vi "subFD_FXP Modeling & Simu.vi"() -> ()   [LabVIEW 2023]
uses:
  <vilib>/addons/Digital Filter Design/_Objects.llb/DFD Filter Obj.ctl
  <vilib>/addons/Digital Filter Design/_Objects.llb/DFD Filter Coef.ctl
  <vilib>/addons/Digital Filter Design/_Objects.llb/DFD Filter Structure Type Selector.ctl
  <vilib>/addons/Digital Filter Design/_Objects.llb/dfd_Internal Quantization Settings.ctl
  <vilib>/addons/Digital Filter Design/_Objects.llb/dfd_Internal Quantization Srcs.ctl
  <vilib>/addons/Digital Filter Design/_Objects.llb/DFD Coef Norm Type.ctl
  <vilib>/addons/Digital Filter Design/_Objects.llb/DFD Quantization Sources.ctl
  <vilib>/addons/Digital Filter Design/_Objects.llb/DFD FXP Statistics Data.ctl
  <vilib>/addons/Digital Filter Design/FXPModel.llb/DFD FXP Get Quantizer (One).vi
  <vilib>/Utility/VariantDataType/GetNumericFxpInfo.vi
  <vilib>/addons/Digital Filter Design/FXPSim.llb/dfd_Check Input FXP Settings.vi
  <vilib>/addons/Digital Filter Design/FXPSim.llb/dfd_Check SRate Simulation Integer Input.vi
  <vilib>/addons/Digital Filter Design/FXPSim.llb/dfd_FXP Simu.vi
  <vilib>/addons/Digital Filter Design/Process.llb/DFD Filtering (Array).vi
  <vilib>/addons/Digital Filter Design/FXPModel.llb/DFD FXP Set Quantizer (One).vi
  <vilib>/addons/Digital Filter Design/FXPModel.llb/DFD FXP Get Quantizer (All).vi
  <vilib>/addons/Digital Filter Design/FilterLib.llb/DFD Save Filter to File.vi
  <vilib>/addons/Digital Filter Design/FXPSim.llb/SimXnode/DFD FXP Simulation.xnode
  <vilib>/addons/Digital Filter Design/NI_DigFilterLicensed.lvlib
  <vilib>/Analysis/NI_AALBase.lvlib
  <vilib>/Analysis/NI_AALPro.lvlib
  <vilib>/addons/Digital Filter Design/NI_DigFilter_FXP.lvlib
  <vilib>/Utility/VariantDataType/VariantType.lvlib
panel:
  in  "Amplitude":dbl=0.99 min=0.0001 max=1.0 step=0.0001
  in  "Random Input":bool
  in  "Frequency":dbl=1000.1 format="%#_5p Hz"
  in  "Pure Sine Input":bool=TRUE
  in  "Save Filter to File":bool
  in  "Run":bool
  in  "Apply default model?":bool=TRUE
  in  "Delay Quantizer":T1={"source"=1, "wl"=16, "iwl"=1, "o-mode"=0, "q_mode"=0, "signed?"=TRUE} {"q_mode" items=["Nearest", "Truncation"]; "o-mode" items=["Saturation", "Wrap"]; "wl" min=1 max=32 step=1; "source" items=["Coefficient", "Input", "Output", "Multiplicand", "Product", "Sum", "Delay"]}
  in  "Sum Quantizer":T1={"source"=1, "wl"=16, "iwl"=1, "o-mode"=0, "q_mode"=0, "signed?"=TRUE} {"q_mode" items=["Nearest", "Truncation"]; "o-mode" items=["Saturation", "Wrap"]; "wl" min=1 max=32 step=1; "source" items=["Coefficient", "Input", "Output", "Multiplicand", "Product", "Sum", "Delay"]}
  in  "Product Quantizer":T1={"source"=1, "wl"=16, "iwl"=1, "o-mode"=0, "q_mode"=0, "signed?"=TRUE} {"q_mode" items=["Nearest", "Truncation"]; "o-mode" items=["Saturation", "Wrap"]; "wl" min=1 max=32 step=1; "source" items=["Coefficient", "Input", "Output", "Multiplicand", "Product", "Sum", "Delay"]}
  in  "Multiplicand Quantizer":T1={"source"=1, "wl"=16, "iwl"=1, "o-mode"=0, "q_mode"=0, "signed?"=TRUE} {"q_mode" items=["Nearest", "Truncation"]; "o-mode" items=["Saturation", "Wrap"]; "wl" min=1 max=32 step=1; "source" items=["Coefficient", "Input", "Output", "Multiplicand", "Product", "Sum", "Delay"]}
  in  "Output Quantizer":T1={"source"=1, "wl"=16, "iwl"=1, "o-mode"=0, "q_mode"=0, "signed?"=TRUE} {"q_mode" items=["Nearest", "Truncation"]; "o-mode" items=["Saturation", "Wrap"]; "wl" min=1 max=32 step=1; "source" items=["Coefficient", "Input", "Output", "Multiplicand", "Product", "Sum", "Delay"]}
  in  "Input Quantizer":T1={"source"=1, "wl"=16, "iwl"=1, "o-mode"=0, "q_mode"=0, "signed?"=TRUE} {"q_mode" items=["Nearest", "Truncation"]; "o-mode" items=["Saturation", "Wrap"]; "wl" min=1 max=32 step=1; "source" items=["Coefficient", "Input", "Output", "Multiplicand", "Product", "Sum", "Delay"]}
  out "modeling":i32(listbox)=6
  out "Simulation Statistics":string="  "
  out "MSE":dbl format="%.3e"
  out "Simulation Results":dbl[][](graph)
  out "Successful Design?":bool
  out "filter out":T2={"mSRate_Fs"=1.0, "mSRate_Version"="1.0", "mSRate_Comments"="", "mSRate_OrgCoef"={"type"=enum."Undefined", "gain"=1.0, "coef a (k)"=[], "coef b (v)"=[]}, "mSRate_CurCoef"={"type"=enum."Undefined", "gain"=1.0, "coef a (k)"=[], "coef b (v)"=[]}, "mSRate_Quantized?"=FALSE, "mSRate_QCoef"={"type"=enum."Undefined", "gain"=1.0, "coef a (k)"=[], "coef b (v)"=[]}, "mSRate_QSettings"=[], "mSRate_Order"=0, "mSRate_Scaling"={"mSRate_ScaleByPowerOf2?"=FALSE, "mSRate_ScaleType"=enum."No Norm"}} {"mSRate_QSettings"."source" items=["Coef a/k"=0, "Coef b/v"=7, "Input"=1, "Output"=2, "Multiplicand"=3, "Product"=4, "Sum"=5, "Delay"=6, "Gain"=8]}
  in  "filter in":T2={"mSRate_Fs"=1.0, "mSRate_Version"="1.0", "mSRate_Comments"="", "mSRate_OrgCoef"={"type"=enum."Undefined", "gain"=1.0, "coef a (k)"=[], "coef b (v)"=[]}, "mSRate_CurCoef"={"type"=enum."Undefined", "gain"=1.0, "coef a (k)"=[], "coef b (v)"=[]}, "mSRate_Quantized?"=FALSE, "mSRate_QCoef"={"type"=enum."Undefined", "gain"=1.0, "coef a (k)"=[], "coef b (v)"=[]}, "mSRate_QSettings"=[], "mSRate_Order"=0, "mSRate_Scaling"={"mSRate_ScaleByPowerOf2?"=FALSE, "mSRate_ScaleType"=enum."No Norm"}} {"mSRate_QSettings"."source" items=["Coef a/k"=0, "Coef b/v"=7, "Input"=1, "Output"=2, "Multiplicand"=3, "Product"=4, "Sum"=5, "Delay"=6, "Gain"=8]}
  out "OK":bool
  in  "stop":bool
  # "Simulation Results"
  # "Simulation Statistics"
  # "Fixed-Point Filter Modeling"
  # "Simulation Source"
  # "Frequency"
  # "Amplitude"
  # "MSE"
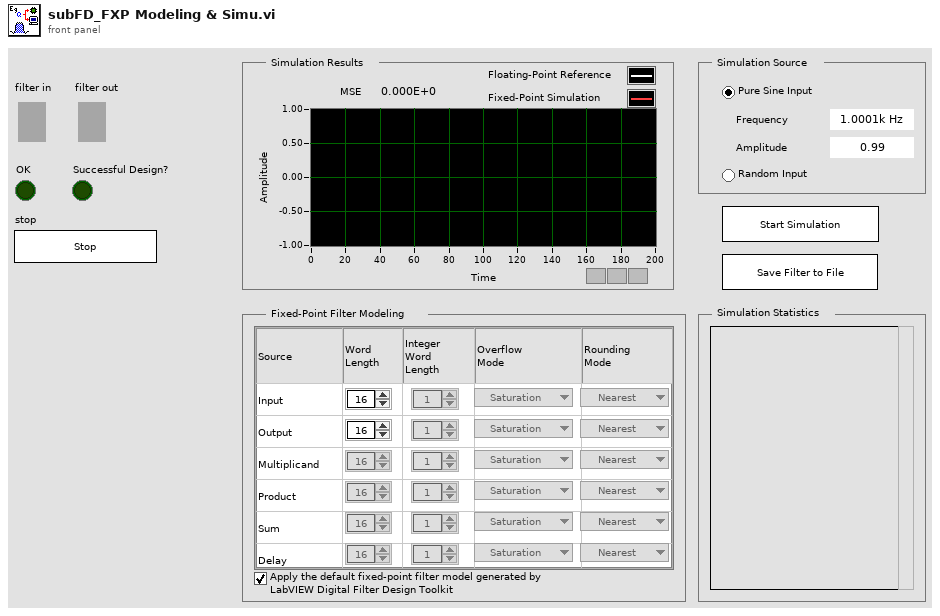
[diagram p1: front panel]
types:
  T1 = cluster{"source":u16, "wl":i16, "iwl":i16, "o-mode":u16, "q_mode":u16, "signed?":bool}
  T2 = typedef "NI_DigFilterLicensed.lvlib/DFD Filter Obj.ctl" = cluster{"mSRate_Fs":dbl, "mSRate_Version":string, "mSRate_Comments":string, "mSRate_OrgCoef":T3, "mSRate_CurCoef":T3, "mSRate_Quantized?":bool, "mSRate_QCoef":T3, "mSRate_QSettings":T5[], "mSRate_Order":i32, "mSRate_Scaling":cluster{"mSRate_ScaleByPowerOf2?":bool, "mSRate_ScaleType":T7}}
  T3 = typedef "NI_DigFilterLicensed.lvlib/DFD Filter Coef.ctl" = cluster{"type":T4, "gain":dbl, "coef a (k)":dbl[], "coef b (v)":dbl[]}
  T4 = typedef "NI_DigFilterLicensed.lvlib/DFD Filter Structure Type Selector.ctl" = enum16{"Undefined", "FIR Direct Form", "FIR Direct Form Transposed", "FIR Symmetric", "FIR Antisymmetric", "IIR Direct Form I", "IIR Direct Form I Transposed", "IIR Direct Form II", "IIR Direct Form II Transposed", "IIR Cascaded Second Order Sections Form I", "IIR Cascaded Second Order Sections Form I Transposed", "IIR Cascaded Second Order Sections Form II", "IIR Cascaded Second Order Sections Form II Transposed", "Lattice Allpass (basic sections)", "Lattice Allpass (one multiplier sections)", "Lattice Allpass (normalized sections)", "Lattice AR (basic sections)", "Lattice AR (one multiplier sections)", "Lattice AR (normalized sections)", "Lattice MA (minimum phase)", "Lattice MA (maximum phase)", "Lattice ARMA (basic sections)", "Lattice ARMA (one multiplier sections)", "Lattice ARMA (normalized sections)"}
  T5 = typedef "NI_DigFilterLicensed.lvlib/dfd_Internal Quantization Settings.ctl" = cluster{"source":T6, "wl":i16, "iwl":i16, "overflow mode":enum16{"Saturation", "Wrap"}, "rounding mode":enum16{"Nearest", "Truncation"}, "signed?":bool}
  T6 = typedef "NI_DigFilterLicensed.lvlib/dfd_Internal Quantization Srcs.ctl" = u16
  T7 = typedef "NI_DigFilterLicensed.lvlib/DFD Coef Norm Type.ctl" = enum16{"No Norm", "Time Domain 1-Norm", "Time Domain 2-Norm", "Time Domain Inf-Norm"}
  T8 = typedef "NI_DigFilterLicensed.lvlib/DFD Quantization Sources.ctl" = u16
  T9 = typedef "NI_DigFilterLicensed.lvlib/DFD FXP Statistics Data.ctl" = cluster{"max value":ext, "min value":ext, "#overflows":i32, "#underflows":i32, "#operations":i32}
  T10 = cluster{"quantizer source":T8, "statistics information":T9}[]
  T11 = typedef "NI_DigFilterLicensed.lvlib/DFD Quantization Settings.ctl" = cluster{"source":T8, "wl":i16, "iwl":i16, "overflow mode":enum16{"Saturation", "Wrap"}, "rounding mode":enum16{"Nearest", "Truncation"}, "signed?":bool}
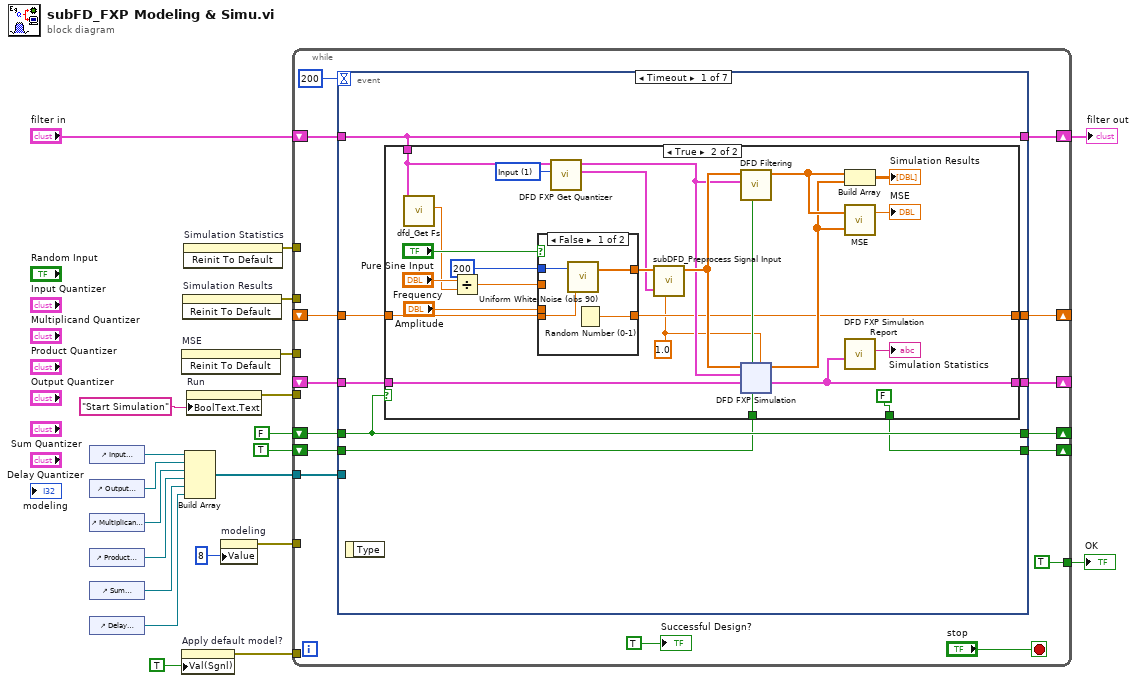
[diagram p0: block diagram]
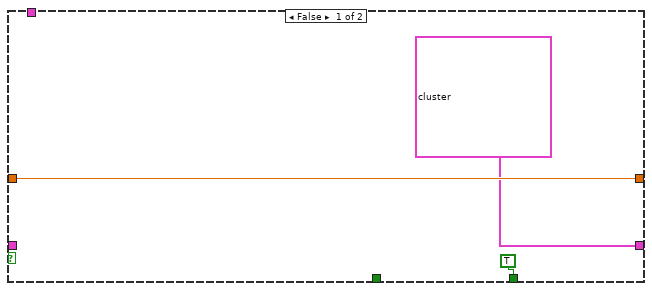
[diagram p2: hidden frame]
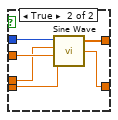
[diagram p3: hidden frame]
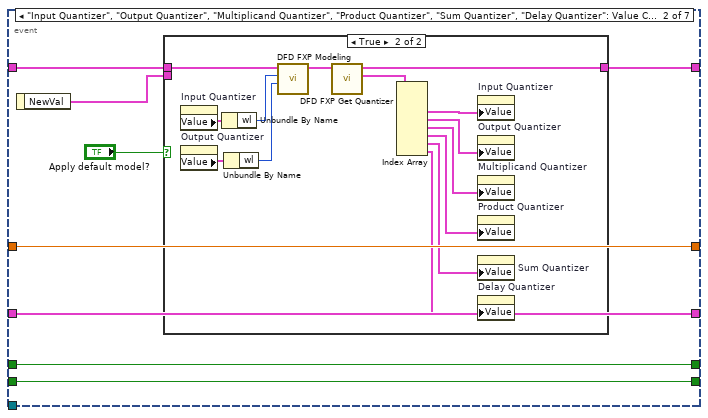
[diagram p4: hidden frame]
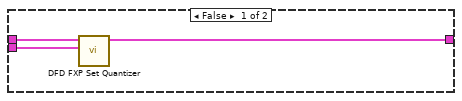
[diagram p5: hidden frame]
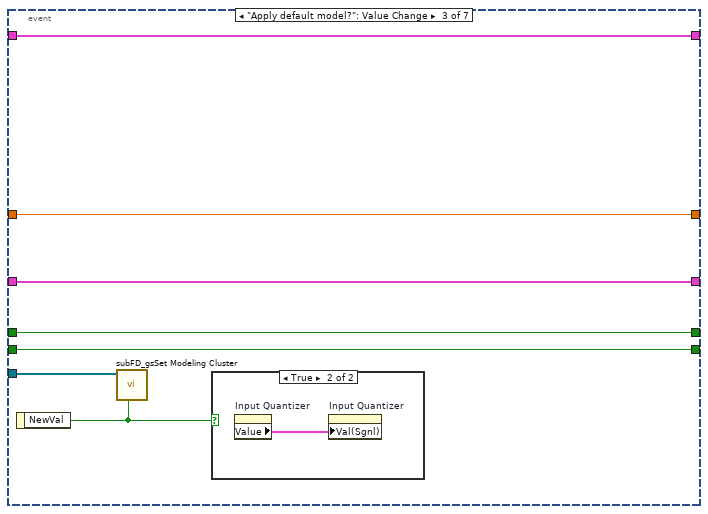
[diagram p6: hidden frame]
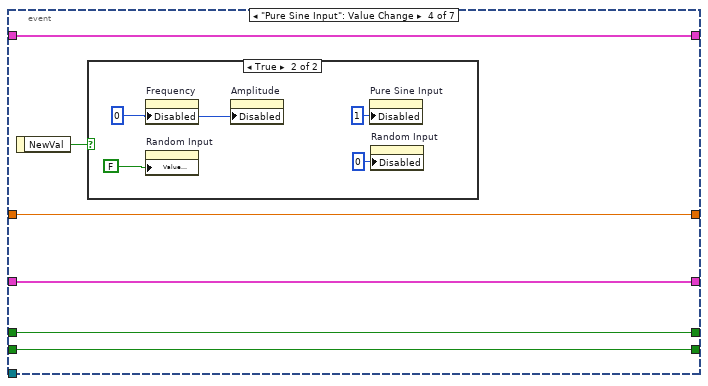
[diagram p8: hidden frame]
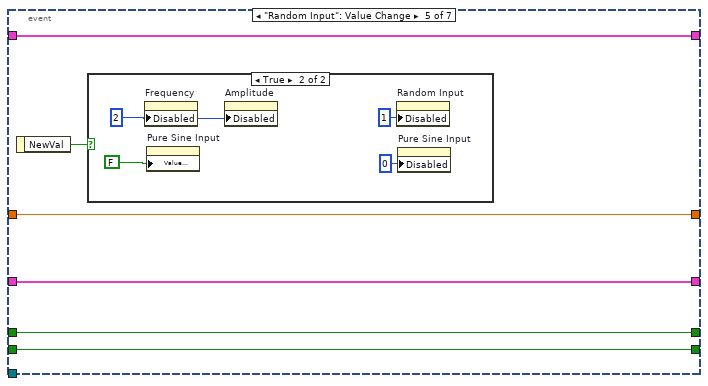
[diagram p10: hidden frame]
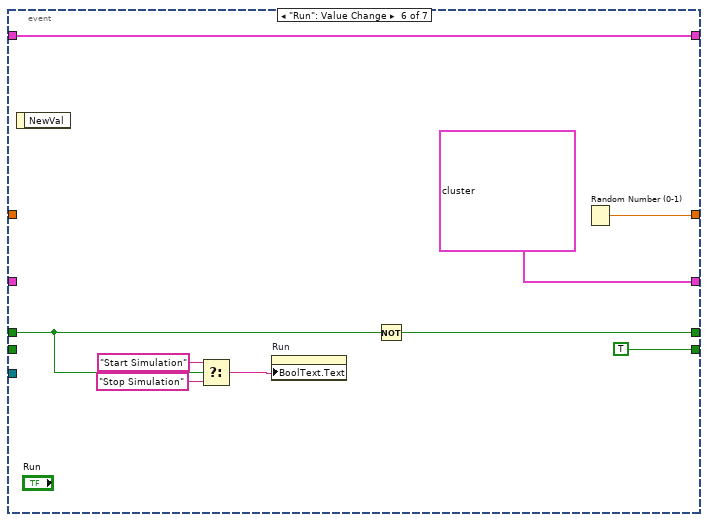
[diagram p12: hidden frame]
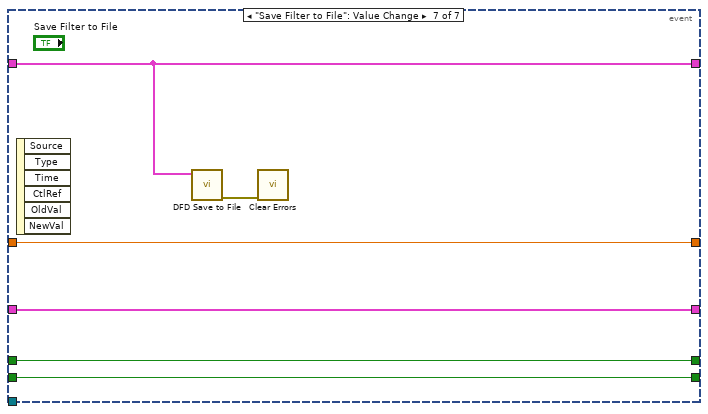
[diagram p13: hidden frame]
diagram:
  n1 = control-ref of="Input Quantizer"() -> (w11:refnum<vi>)
  n2 = control-ref of="Output Quantizer"() -> (w12:refnum<vi>)
  n3 = control-ref of="Multiplicand Quantizer"() -> (w17:refnum<vi>)
  n4 = control-ref of="Product Quantizer"() -> (w16:refnum<vi>)
  n5 = control-ref of="Sum Quantizer"() -> (w15:refnum<vi>)
  n6 = control-ref of="Delay Quantizer"() -> (w14:refnum<vi>)
  n7 = invoke on="MSE" class="DigNum (strict)" method="Reinit To Default"() -> (error out=w7:errorcluster)  [unwired: 3 in, 2 out]
  n8 = property on="Apply default model?" class="Bool (strict)"("Val(Sgnl)"=TRUE ("auto?")) -> (error out=w8:errorcluster)  [unwired: 2 in, 1 out]
  n9 = invoke on="Simulation Results" class="WFGraph (strict)" method="Reinit To Default"() -> (error out=w6:errorcluster)  [unwired: 3 in, 2 out]
  n10 = invoke on="Simulation Statistics" class="Str" method="Reinit To Default"() -> (error out=w5:errorcluster)  [unwired: 3 in, 2 out]
  n11 = Build Array(w11, w12, w17, w16, w15, w14) -> (w13:refnum<vi>[])
  n12 = property on="Run" class="Bool"("BoolText.Text"="Start Simulation" ("t")) -> (error out=w4:errorcluster)  [unwired: 2 in, 1 out]
  n13 = property on="modeling" class="MCListbox (strict)"("Value"=8) -> (error out=w18:errorcluster)  [unwired: 2 in, 1 out]
  n14 = while {
    tunnel: [TRUE] -> w21
    shift-right: [w32] -> w20
    shift-left: "filter in" -> [w33]
    tunnel: w18 -> [_]
    tunnel: w13 -> [w30]
    shift-right: [w28] -> _
    shift-left: FALSE -> [w29]
    tunnel: w8 -> [_]
    tunnel: w7 -> [_]
    tunnel: w6 -> [_]
    tunnel: w5 -> [_]
    tunnel: w4 -> [_]
    shift-right: [w26] -> _
    shift-left: TRUE -> [w27]
    shift-right: [w25] -> _
    shift-left: _ -> [w24]
    shift-right: [w23] -> _
    shift-left: _ -> [w22]
    stop <- "stop" stop-if-true
    n15 = event shown="[0] Timeout" {
      selector: _ -> [_ _ _ _ _ _ _]
      dyn-events: _ -> [_ _ _ _ _ _ _]
      timeout: 200 -> [_ _ _ _ _ _ _]
      tunnel: w33 -> [w42 w122 w146 w152 w162 w176 w182]
      tunnel: [w42 w118 w146 w152 w162 w176 w182] -> w32
      tunnel: w30 -> [_ _ w144 _ _ _ _]
      tunnel: w29 -> [w44 w119 w143 w151 w161 w174 w180]
      tunnel: [w44 w119 w143 w151 w161 w175 w180] -> w28
      tunnel: w27 -> [w43 w115 w140 w148 w158 _ w179]
      tunnel: [w41 w115 w140 w148 w158 TRUE w179] -> w26
      tunnel: [w40 w116 w141 w149 w159 T10 [{"quantizer source"=0, "statistics information"={"max value"=-inf, "min value"=inf, "#overflows"=0, "#underflows"=0, "#operations"=0}}, {"quantizer source"=1, "statistics information"={"max value"=-inf, "min value"=inf, "#overflows"=0, "#underflows"=0, "#operations"=0}}, {"quantizer source"=2, "statistics information"={"max value"=-inf, "min value"=inf, "#overflows"=0, "#underflows"=0, "#operations"=0}}, {"quantizer source"=3, "statistics information"={"max value"=-inf, "min value"=inf, "#overflows"=0, "#underflows"=0, "#operations"=0}}, {"quantizer source"=4, "statistics information"={"max value"=-inf, "min value"=inf, "#overflows"=0, "#underflows"=0, "#operations"=0}}, {"quantizer source"=5, "statistics information"={"max value"=-inf, "min value"=inf, "#overflows"=0, "#underflows"=0, "#operations"=0}}, {"quantizer source"=6, "statistics information"={"max value"=-inf, "min value"=inf, "#overflows"=0, "#underflows"=0, "#operations"=0}}] ("filtering statistics in") w178] -> w25
      tunnel: w24 -> [w39 w116 w141 w149 w159 _ w178]
      tunnel: [w38 w117 w142 w150 w160 w170 w177] -> w23
      tunnel: w22 -> [w37 w117 w142 w150 w160 _ w177]
      event Timeout {
        n16 = event-data() -> ()  [unwired: 2 out]
        n17 = case shown="True" w44 {
          tunnel: w43 -> [_ w59]
          tunnel: w42 -> [_ w58]
          tunnel: [TRUE FALSE] -> w41
          tunnel: [T10 [{"quantizer source"=0, "statistics information"={"max value"=-inf, "min value"=inf, "#overflows"=0, "#underflows"=0, "#operations"=0}}, {"quantizer source"=1, "statistics information"={"max value"=-inf, "min value"=inf, "#overflows"=0, "#underflows"=0, "#operations"=0}}, {"quantizer source"=2, "statistics information"={"max value"=-inf, "min value"=inf, "#overflows"=0, "#underflows"=0, "#operations"=0}}, {"quantizer source"=3, "statistics information"={"max value"=-inf, "min value"=inf, "#overflows"=0, "#underflows"=0, "#operations"=0}}, {"quantizer source"=4, "statistics information"={"max value"=-inf, "min value"=inf, "#overflows"=0, "#underflows"=0, "#operations"=0}}, {"quantizer source"=5, "statistics information"={"max value"=-inf, "min value"=inf, "#overflows"=0, "#underflows"=0, "#operations"=0}}, {"quantizer source"=6, "statistics information"={"max value"=-inf, "min value"=inf, "#overflows"=0, "#underflows"=0, "#operations"=0}}] ("filtering statistics in") w55] -> w40
          tunnel: w39 -> [_ w54]
          tunnel: [w46 w52] -> w38
          tunnel: w37 -> [w46 w51]
          frame False {
          }
          frame True {
            w48 = 1.0 ("amp")
            w62 = T8 1 items=["Coefficients a/k"=0, "Coefficients b/v"=7, "Input"=1, "Output"=2, "Multiplicand"=3, "Product"=4, "Sum"=5, "Delay"=6] ("quantizer source")
            n18 = call <vilib>:"dfd_Get Fs.vi"("filter in"=w58) -> ("fs [Hz]"=w49:dbl)  [unwired: 1 in, 9 out]
            n19 = Divide(x="Frequency", y=w49) -> (x/y=w69:dbl)
            n20 = case shown="False" "Pure Sine Input" {
              tunnel: w69 -> [_ w114]
              tunnel: [w108 w113] -> w64
              tunnel: 200 -> [w107 w112]
              tunnel: [w105 w111] -> w52
              tunnel: w51 -> [w106 w110]
              tunnel: "Amplitude" -> [_ w109]
              frame False {
                n21 = call <vilib>:"Uniform White Noise (obs 90).vi"("seed"=w106, "samples"=w107) -> ("uniform white noise"=w108:dbl[])  [unwired: 1 in, 1 out]
                n22 = Random Number (0-1)() -> (number: 0 to 1=w105:dbl)
              }
              frame True {
                n23 = call <vilib>:"Sine Wave.vi"("samples"=w112, "amplitude"=w109, "frequency"=w114, "phase in"=w110) -> ("sine wave"=w113:dbl[], "phase out"=w111:dbl)  [unwired: 1 in, 1 out]
              }
            }
            n24 = call-poly <vilib>:"DFD FXP Get Quantizer.vi"("quantizer source"=w62, "filter in"=w58) -> ("quantizer"=w61:T11, "filter out"=w57:T2)  [unwired: 1 in, 7 out]
            n25 = call <vilib>:"subDFD_Preprocess Signal Input.vi"("input quantizer"=w61, "input range"=w48, "x"=w64) -> ("q[x]"=w63:dbl[])  [unwired: 8 out]
            n26 = call-poly <vilib>:"DFD Filtering.vi"("init? (F)"=w59, "filter"=w57, "signal in"=w63) -> ("signal out"=w66:dbl[])  [unwired: 1 in, 7 out]
            n27 = xnode "DFD FXP Simulation"("input range"=w48, "init? (T)"=w59, "filtering statistics in"=w54, "filter in"=w57, "signal in"=w63) -> ("filtering statistics report"=w55:T10, "DBL signal out"=w60:dbl[])  [unwired: 1 in, 2 out]
            n28 = Build Array(w66, w60) -> (→"Simulation Results":dbl[][])
            n29 = call <vilib>:"MSE.vi"("X Values"=w60, "Y Values"=w66) -> ("mse"=→"MSE":dbl)  [unwired: 1 out]
            n30 = call <vilib>:"DFD FXP Simulation Report.vi"("filtering statistics report"=w55) -> ("filtering text report"=→"Simulation Statistics":string)  [unwired: 1 in, 9 out]
          }
        }
      }
      event "Input Quantizer", "Output Quantizer", "Multiplicand Quantizer", "Product Quantizer", "Sum Quantizer", "Delay Quantizer": Value Change {
        n31 = event-data() -> ("NewVal"=w121:T1)  [unwired: 1 out]
        n32 = case shown="True" "Apply default model?" {
          tunnel: w122 -> [w125 w139]
          tunnel: w121 -> [w124 _]
          tunnel: [w123 w128] -> w118
          frame False {
            n33 = call-poly <vilib>:"DFD FXP Set Quantizer.vi"("quantizer"=w124, "filter in"=w125) -> ("filter out"=w123:T2)  [unwired: 1 in, 8 out]
          }
          frame True {
            n34 = property on="Input Quantizer" class="Clust (strict)"() -> ("Value"=w138:T1)  [unwired: 2 in, 2 out]
            n35 = property on="Output Quantizer" class="Clust (strict)"() -> ("Value"=w137:T1)  [unwired: 2 in, 2 out]
            n36 = Unbundle By Name(w138) -> ("wl"=w136:i16)
            n37 = Unbundle By Name(w137) -> ("wl"=w135:i16)
            n38 = call <vilib>:"DFD FXP Modeling.vi"("output word length"=w135, "input word length"=w136, "filter in"=w139) -> ("filter out"=w129:T2)  [unwired: 4 in, 4 out]
            n39 = call-poly <vilib>:"DFD FXP Get Quantizer.vi"("filter in"=w129) -> ("quantizers"=w127:T11[], "filter out"=w128:T2)  [unwired: 1 in, 8 out]
            n40 = Index Array(array=w127) -> (element #2=w134:T11, element #3=w133:T11, element #4=w132:T11, element #5=w131:T11, element #6=w130:T11, element #7=w126:T11)  [unwired: 7 in, 1 out]
            n41 = property on="Input Quantizer" class="Clust (strict)"("Value"=w134) -> ()  [unwired: 2 in, 2 out]
            n42 = property on="Output Quantizer" class="Clust (strict)"("Value"=w133) -> ()  [unwired: 2 in, 2 out]
            n43 = property on="Multiplicand Quantizer" class="Clust (strict)"("Value"=w132) -> ()  [unwired: 2 in, 2 out]
            n44 = property on="Product Quantizer" class="Clust (strict)"("Value"=w131) -> ()  [unwired: 2 in, 2 out]
            n45 = property on="Sum Quantizer" class="Clust (strict)"("Value"=w130) -> ()  [unwired: 2 in, 2 out]
            n46 = property on="Delay Quantizer" class="Clust (strict)"("Value"=w126) -> ()  [unwired: 2 in, 2 out]
          }
        }
      }
      event "Apply default model?": Value Change {
        n47 = event-data() -> ("NewVal"=w145:bool)  [unwired: 1 out]
        n48 = call "subFD_gsSet Modeling Cluster.vi"("auto?"=w145, "Cluster group1"=w144) -> ()  [unwired: 1 in, 9 out]
        n49 = case shown="True" w145 {
          frame False {
          }
          frame True {
            n50 = property on="Input Quantizer" class="Clust (strict)"() -> ("Value"=w147:T1)  [unwired: 2 in, 2 out]
            n51 = property on="Input Quantizer" class="Clust (strict)"("Val(Sgnl)"=w147) -> ()  [unwired: 2 in, 2 out]
          }
        }
      }
      event "Pure Sine Input": Value Change {
        n52 = event-data() -> ("NewVal"=w153:bool)  [unwired: 1 out]
        n53 = case shown="True" w153 {
          frame False {
          }
          frame True {
            w154 = u8 0 ("Disabled")
            n54 = property on="Frequency" class="DigNum (strict)"("Disabled"=w154) -> ()  [unwired: 2 in, 2 out]
            n55 = property on="Random Input" class="Bool (strict)"("Value (Signaling)"=FALSE) -> ()  [unwired: 2 in, 2 out]
            n56 = property on="Amplitude" class="DigNum (strict)"("Disabled"=w154) -> ()  [unwired: 2 in, 2 out]
            n57 = property on="Pure Sine Input" class="Bool (strict)"("Disabled"=u8 1) -> ()  [unwired: 2 in, 2 out]
            n58 = property on="Random Input" class="Bool (strict)"("Disabled"=u8 0) -> ()  [unwired: 2 in, 2 out]
          }
        }
      }
      event "Random Input": Value Change {
        n59 = event-data() -> ("NewVal"=w163:bool)  [unwired: 1 out]
        n60 = case shown="True" w163 {
          frame False {
          }
          frame True {
            w164 = u8 2 ("Disabled")
            n61 = property on="Frequency" class="DigNum (strict)"("Disabled"=w164) -> ()  [unwired: 2 in, 2 out]
            n62 = property on="Pure Sine Input" class="Bool (strict)"("Value (Signaling)"=FALSE) -> ()  [unwired: 2 in, 2 out]
            n63 = property on="Amplitude" class="DigNum (strict)"("Disabled"=w164) -> ()  [unwired: 2 in, 2 out]
            n64 = property on="Random Input" class="Bool (strict)"("Disabled"=u8 1) -> ()  [unwired: 2 in, 2 out]
            n65 = property on="Pure Sine Input" class="Bool (strict)"("Disabled"=u8 0) -> ()  [unwired: 2 in, 2 out]
          }
        }
      }
      event "Run": Value Change {
        n66 = event-data() -> ()  [unwired: 2 out]
        n67 = Select(t="Start Simulation", s=w174, f="Stop Simulation") -> (s? t:f=w171:string)
        n68 = property on="Run" class="Bool"("BoolText.Text"=w171) -> ()  [unwired: 2 in, 2 out]
        n69 = Not(x=w174) -> (.not. x?=w175:bool)
        n70 = Random Number (0-1)() -> (number: 0 to 1=w170:dbl)
      }
      event "Save Filter to File": Value Change {
        n71 = event-data() -> ()  [unwired: 7 out]
        n72 = call-poly <vilib>:"DFD Save to File.vi"("filter in"=w182) -> ("error out"=w181:errorcluster)  [unwired: 3 in, 7 out]
        n73 = call <vilib>:"Clear Errors.vi"("error in (no error)"=w181) -> ()  [unwired: 1 in, 6 out]
      }
    }
    "Successful Design?" <- TRUE ("Successful Design?")
  }
  "OK" <- w21
  "filter out" <- w20
